vi "JSON Config Performance Test.vi"() -> ()   [LabVIEW 2021]
uses:
  <vilib>/Platform/TimedLoop/XDataNode/timing_clust.ctl
  <vilib>/Platform/TimedLoop/XDataNode/nitl_modes.ctl
  <vilib>/Platform/TimedLoop/XDataNode/wakeup.ctl
  OOB_Rx/CIFCoreOOB_Rx.lvclass/CIFCoreOOB_Rx.ctl
  CIFUtilities/CIFOutOfBand/CIFOutOfBand.lvclass/CIFOutOfBand.ctl
  OOB_Rx/Private/Command Settings.vi
  CIFUtilities/CIFOutOfBand/Accessors/Write Local OOB Data.vi
  CIFUtilities/CIFOutOfBand/Accessors/Read Local OOB Data.vi
  CIFUtilities/CIFOutOfBand/Write OOB DVR.vi
  CIFUtilities/CIFOutOfBand/Utilities/Command to Bitwise Command.vi
  CIFUtilities/CIFOutOfBand/Read OOB DVR.vi
  OOB_Rx/Private/Read Payload.vi
  OOB_Rx/CIFCoreOOB_Rx.lvclass
  D:/dev/CIF-LVCore/src/CIFUtilities/CIFOutOfBand/CIFOutOfBand.lvclass
  CIFUtilities/CIFOutOfBand/Init OOB.vi
  <vilib>/addons/_JKI.lib/Serialization/JSON/Library/Unflatten From JSON String.vi
  <vilib>/Platform/TimedLoop/XDataNode/XDataNode.xnode
  <vilib>/addons/_JKI.lib/Serialization/JSON/JKI JSON Serialization.lvlib
  <vilib>/Platform/TimedLoop/XDataNode/XDNodeRunTimeDep.lvlib
  CIFUtilities/CIFOutOfBand/CIFOutOfBand.lvclass
panel:
  out "Max":dbl
  out "avg":dbl
  out "pass":bool
  out "error out":errorcluster
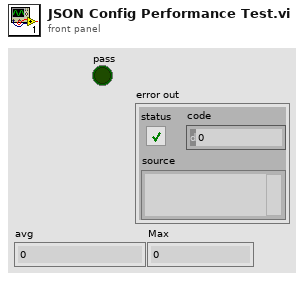
[diagram p1: front panel]
types:
  T1 = cluster{"Numeric":dbl, "Array":cluster{"Numeric":dbl, "String":string, "Boolean":bool}[], "string":string, "Null array":u8[]}
  T2 = typedef "XDNodeRunTimeDep.lvlib/timing_clust.ctl" = cluster{"Expected End [f-1]":u64, "Actual End [f-1]":u64, "Finished Late? [f-1]":bool, "Expected End [i-1]":u64, "Actual End [i-1]":u64, "Finished Late? [i-1]":bool, "Expected Start [i]":u64, "Actual Start [i]":u64, "Expected Start [f]":u64, "Actual Start [f]":u64, "Source Name":string, "Structure Name":string, "Period":i64, "Deadline":i64, "Offset":i64, "Start":i64, "Priority":i32, "Timeout":i32, "Mode":T3, "Wakeup Reason":T4, "Error":errorcluster, "Source Type":string, "Secondary Source Type":string, "Global End Time":u64, "Global Start Time":u64, "Frame Duration":u64, "Iteration Duration":u64, "Assigned CPU":i32, "I/O Scan Engine Mode":u32}
  T3 = typedef "XDNodeRunTimeDep.lvlib/nitl_modes.ctl" = enum32{"No Change", "Process missed periods, maintain original phase", "Discard missed periods, maintain original phase", "Process missed periods, ignore original phase", "Discard missed periods, ignore original phase"}
  T4 = typedef "XDNodeRunTimeDep.lvlib/wakeup.ctl" = enum32{"Normal", "Aborted", "Asynchronous wakeup", "Timing source error", "Timed loop error", "Timeout"}
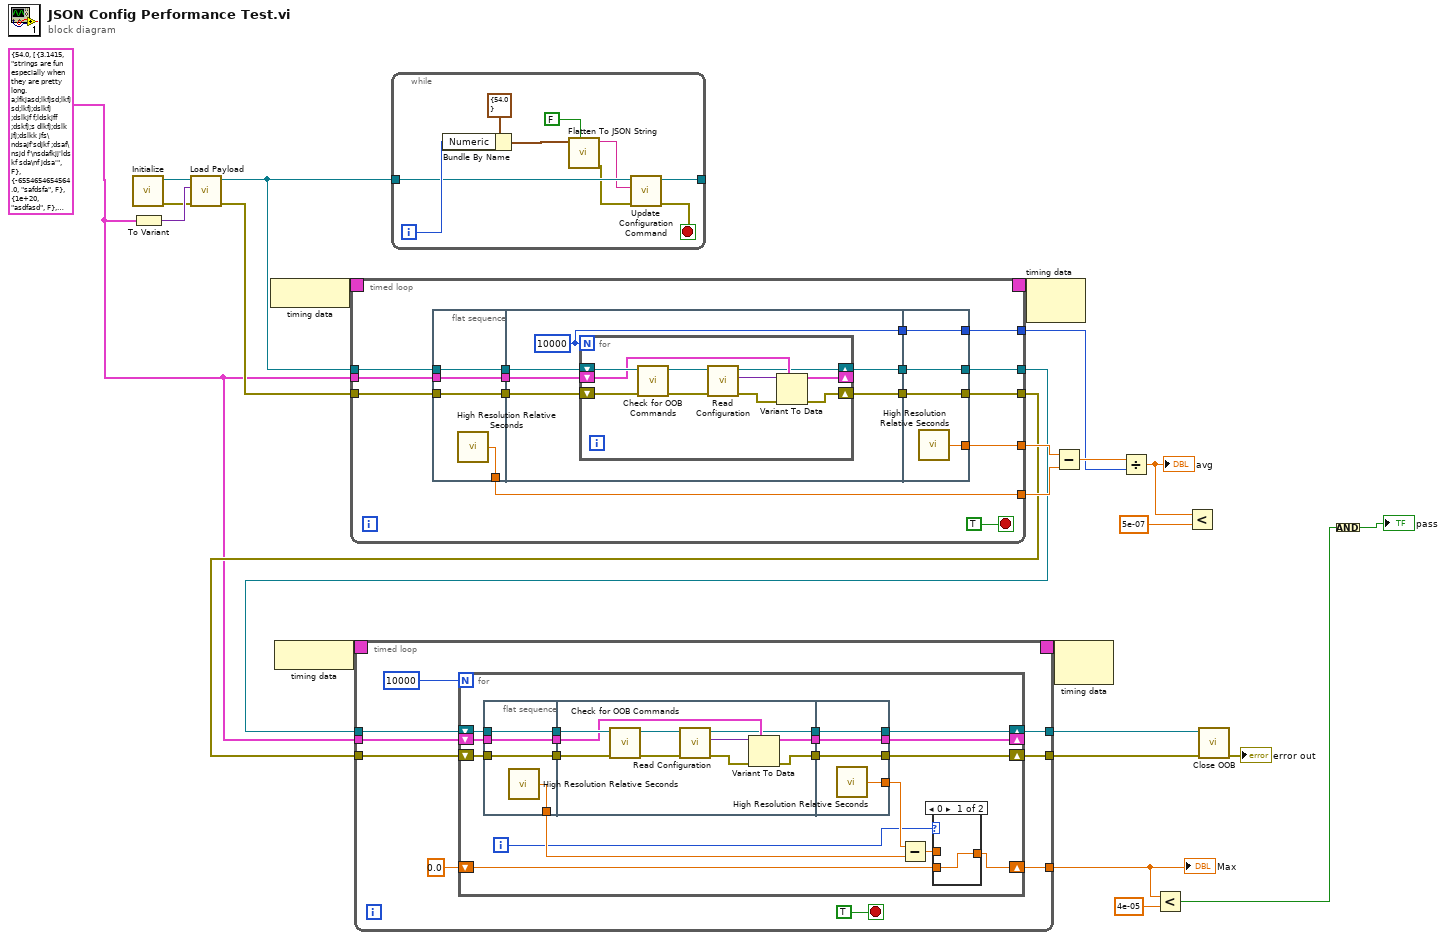
[diagram p0: block diagram]
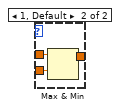
[diagram p2: hidden frame]
diagram:
  w4 = T1 {"Numeric"=54.0, "Array"=[{"Numeric"=3.1415, "String"="strings are fun especially when they are pretty long. a;lfkjasd;lkfjsd;lkfjsd;lkfj;dslkfj ;dslkjf f;ldskjff ;dskfj;s dlkfj;dslk jfj;dslkk jfs\ndsajf'sdjkf ;dsaf\nsjd f'\nsdafkjj'lds kf sda\nf jdsa'", "Boolean"=FALSE}, {"Numeric"=-6554654654564.0, "String"="safdsfa", "Boolean"=FALSE}, {"Numeric"=1e+20, "String"="asdfasd", "Boolean"=FALSE}, {"Numeric"=2.0, "String"="afd", "Boolean"=TRUE}, {"Numeric"=12.34, "String"="data", "Boolean"=FALSE}], "string"="strings", "Null array"=[0]} ("Test Config")
  n1 = call "Initialize.vi"() -> ("error out"=w8:errorcluster, "CoreOOB_Rx out"=w7:refnum<class "CIFCoreOOB_Rx.lvclass">)  [unwired: 10 in]
  n2 = To Variant(anything=w4) -> (Variant=w9:variant)
  n3 = call "Load Payload.vi"("error in (no error)"=w8, "Configuration Payload"=w9, "CoreOOB_Rx in"=w7) -> ("error out"=w5:errorcluster, "CoreOOB_Rx out"=w6:refnum<class "CIFCoreOOB_Rx.lvclass">)  [unwired: 7 in]
  n4 = node-c288() -> (w25:T2)
  n5 = node-c288() -> (w19:T2)
  n6 = timed-loop {
    timing: w25 -> [_]
    timing-out: [_] -> w24
    tunnel: w6 -> [w40]
    tunnel: w5 -> [w39]
    tunnel: [w35] -> w17
    tunnel: [w33] -> w16
    tunnel: [w31] -> w23
    tunnel: [w30] -> w22
    tunnel: [w29] -> w20
    tunnel: w4 -> [w27]
    stop <- TRUE stop-if-true
    n7 = flat-sequence {
      tunnel: w39 -> [w43]
      tunnel: w40 -> [w44]
      tunnel: [w44] -> w37
      tunnel: [w43] -> w36
      tunnel: [w42] -> w30
      tunnel: w27 -> [w41]
      tunnel: [w41] -> w26
      tunnel: w37 -> [w50]
      tunnel: w36 -> [w49]
      tunnel: [w48] -> w34
      tunnel: [w47] -> w32
      tunnel: [w46] -> w28
      tunnel: w26 -> [w45]
      tunnel: [w64] -> w35
      tunnel: w34 -> [w64]
      tunnel: [w63] -> w33
      tunnel: w32 -> [w63]
      tunnel: [w62] -> w31
      tunnel: [w61] -> w29
      tunnel: w28 -> [w61]
      frame #0 {
        n8 = call <vilib>:"High Resolution Relative Seconds.vi"() -> ("relative seconds"=w42:dbl)
      }
      frame #1 {
        w46 = 10000
        n9 = for {
          N: w46 -> [_]
          shift-right: [w53] -> w48
          shift-left: w50 -> [w56]
          shift-right: [w51] -> w47
          shift-left: w49 -> [w54]
          shift-right: [w52] -> _
          shift-left: w45 -> [w55]
          n10 = call "Check for OOB Commands.vi"("error in (no error)"=w54, "CoreOOB_Rx in"=w56) -> ("error out"=w60:errorcluster, "CoreOOB_Rx out"=w57:refnum<class "CIFCoreOOB_Rx.lvclass">)  [unwired: 6 in, 2 out]
          n11 = call "Read Configuration.vi"("error in"=w60, "CoreOOB_Rx in"=w57) -> ("error out"=w58:errorcluster, "Configuration Data"=w59:variant, "CoreOOB_Rx out"=w53:refnum<class "CIFCoreOOB_Rx.lvclass">)  [unwired: 7 in]
          n12 = Variant To Data(error in=w58, type=w55, Variant=w59) -> (data=w52:T1, error out=w51:errorcluster)
        }
      }
      frame #2 {
        n13 = call <vilib>:"High Resolution Relative Seconds.vi"() -> ("relative seconds"=w62:dbl)
      }
    }
  }
  n14 = timed-loop {
    timing: w19 -> [_]
    timing-out: [_] -> w18
    tunnel: w17 -> [w75]
    tunnel: w16 -> [w74]
    tunnel: [w72] -> w3
    tunnel: [w71] -> w2
    tunnel: w4 -> [w70]
    tunnel: [w67] -> w13
    stop <- TRUE stop-if-true
    n15 = for {
      N: 10000 -> [_]
      shift-right: [w87] -> w72
      shift-left: w75 -> [w89]
      shift-right: [w86] -> w71
      shift-left: w74 -> [w88]
      shift-right: [w80] -> w67
      shift-left: 0.0 -> [w81]
      shift-right: [w79] -> _
      shift-left: w70 -> [w85]
      i -> [w77]
      n16 = flat-sequence {
        tunnel: w88 -> [w100]
        tunnel: w89 -> [w101]
        tunnel: [w101] -> w93
        tunnel: [w100] -> w92
        tunnel: [w99] -> w83
        tunnel: w85 -> [w98]
        tunnel: [w98] -> w91
        tunnel: w93 -> [w107]
        tunnel: w92 -> [w105]
        tunnel: [w104] -> w90
        tunnel: w91 -> [w106]
        tunnel: [w102] -> w78
        tunnel: [w103] -> w76
        tunnel: [w115] -> w87
        tunnel: w90 -> [w115]
        tunnel: [w114] -> w86
        tunnel: [w113] -> w84
        tunnel: [w112] -> w79
        tunnel: w78 -> [w112]
        tunnel: w76 -> [w114]
        frame #0 {
          n17 = call <vilib>:"High Resolution Relative Seconds.vi"() -> ("relative seconds"=w99:dbl)
        }
        frame #1 {
          n18 = call "Check for OOB Commands.vi"("error in (no error)"=w105, "CoreOOB_Rx in"=w107) -> ("error out"=w108:errorcluster, "CoreOOB_Rx out"=w111:refnum<class "CIFCoreOOB_Rx.lvclass">)  [unwired: 6 in, 2 out]
          n19 = call "Read Configuration.vi"("error in"=w108, "CoreOOB_Rx in"=w111) -> ("error out"=w110:errorcluster, "Configuration Data"=w109:variant, "CoreOOB_Rx out"=w104:refnum<class "CIFCoreOOB_Rx.lvclass">)  [unwired: 7 in]
          n20 = Variant To Data(error in=w110, type=w106, Variant=w109) -> (data=w102:T1, error out=w103:errorcluster)
        }
        frame #2 {
          n21 = call <vilib>:"High Resolution Relative Seconds.vi"() -> ("relative seconds"=w113:dbl)
        }
      }
      n22 = Subtract(x=w84, y=w83) -> (x-y=w82:dbl)
      n23 = case shown="0" w77 {
        tunnel: w82 -> [_ w97]
        tunnel: w81 -> [w94 w96]
        tunnel: [w94 w95] -> w80
        frame 0 {
        }
        frame 1, Default {
          n24 = Max & Min(x=w97, y=w96) -> (max(x,y)=w95:dbl)  [unwired: 1 out]
        }
      }
    }
  }
  "Max" <- w13
  n25 = while {
    tunnel: [w120] -> _
    tunnel: w6 -> [w122]
    i -> [w123]
    stop <- w119 stop-if-true
    n26 = Bundle By Name(cluster=cluster{"Numeric":dbl} {"Numeric"=54.0} ("Test Config"), "Numeric"=w123) -> (w124:cluster{"Numeric":dbl})
    n27 = call <vilib>:"Flatten To JSON String.vi"("Multiline (T)"=FALSE, "Variant"=w124) -> ("error out"=w118:errorcluster, "JSON String"=w121:string)  [unwired: 8 in]
    n28 = call "Update Configuration Command.vi"("error in"=w118, "Config JSON"=w121, "CoreOOB_Rx in"=w122) -> ("error out"=w119:errorcluster, "CoreOOB_Rx out"=w120:refnum<class "CIFCoreOOB_Rx.lvclass">)  [unwired: 7 in]
  }
  n29 = node-c288(w24) -> ()  [unwired: 1 out]
  n30 = Subtract(x=w23, y=w22) -> (x-y=w21:dbl)
  n31 = node-c288(w18) -> ()  [unwired: 1 out]
  n32 = Divide(x=w21, y=w20) -> (x/y=w15:dbl)
  "avg" <- w15
  n33 = Less?(x=w13, y=4e-05) -> (x < y?=w11:bool)
  n34 = Less?(x=w15, y=5e-07) -> ()  [unwired: 1 out]
  n35 = call "Close OOB.vi"("error in"=w2, "OOB in"=w3) -> ("error out"=→"error out":errorcluster)  [unwired: 9 in]
  n36 = Compound Arithmetic op=AND(w11) -> (→"pass":bool)
